vi "Unregister and Close Sessions.vi"(8 "error in":errorcluster) -> (0 "error out":errorcluster)   [LabVIEW 2020, in "VISA Measurement.lvlib"]
uses:
  VISA Measurement.lvlib
  <vilib>/MeasurementLink/MeasurementLink Session Management V1/Session Reservation/Initialize and Close Session Behavior.ctl
  <vilib>/MeasurementLink/MeasurementLink VISA/Initialize Sessions - NSess.vi
  <vilib>/MeasurementLink/MeasurementLink VISA/MeasurementLink VISA.lvlib
  <vilib>/MeasurementLink/MeasurementLink Session Management V1/Session Reservation/Session Reservation.lvclass
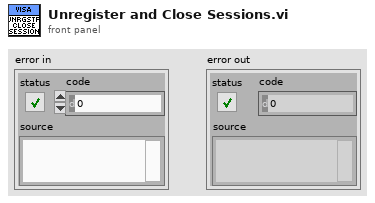
[diagram p1: front panel]
types:
  T1 = typedef "MeasurementLink Session Management V1.lvlib/Session Reservation.lvclass/Initialize and Close Session Behavior.ctl" = enum16{"Auto", "Initialize and Close", "Attach and Detach", "Initialize and Detach", "Attach and Close"}
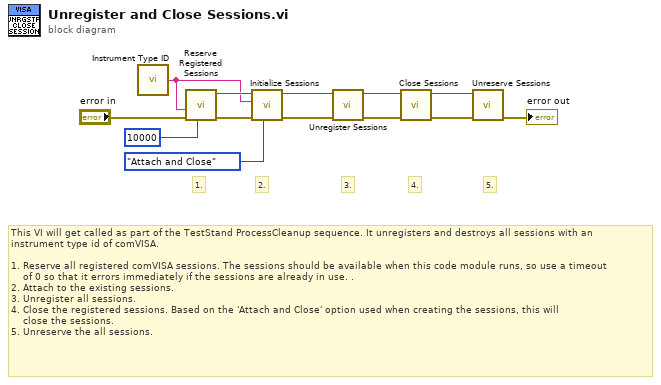
[diagram p0: block diagram]
diagram:
  # "3."
  # "5."
  # "4."
  # "2."
  # "1."
  # "This VI will get called as part of the TestStand ProcessCleanup sequence. It unregisters and destroys all sessions with an \ninstrument type id of comVISA.\n\n1. Reserve all registered comVISA sessions. The sessions should be available when this code module runs, so use a timeout\n    of 0 so that it errors immediately if the sessions are already in use. .\n2. Attach to the existing sessions.\n3. Unregister all sessions.\n4. Close the registered sessions. Based on the 'Attach and Close' option used when creating the sessions, this will\n    close the sessions.\n5. Unreserve the all sessions."
  n1 = call "Instrument Type ID.vi"() -> ("instrument type id"=w2:string)  [unwired: 5 in]
  n2 = call <vilib>:"Reserve Registered Sessions.vi"("timeout (ms)"=10000, "error in"="error in", "instrument type id"=w2) -> ("error out"=w11:errorcluster, "session reservation out"=w10:refnum<class "Session Reservation.lvclass">)  [unwired: 7 in]
  n3 = call-poly <vilib>:"Initialize Sessions.vi"("initialize and close session behavior"=Initialize_and_Close_Session_Behavior."Attach and Close", "error in"=w11, "instrument type id"=w2, "session reservation in"=w10) -> ("error out"=w7:errorcluster, "session reservation out"=w9:refnum<class "Session Reservation.lvclass">)  [unwired: 4 in, 2 out]
  n4 = call <vilib>:"Unregister Sessions.vi"("error in"=w7, "session reservation in"=w9) -> ("error out"=w4:errorcluster, "session reservation out"=w6:refnum<class "Session Reservation.lvclass">)  [unwired: 8 in]
  n5 = call <vilib>:"Close Sessions.vi"("error in"=w4, "session reservation in"=w6) -> ("error out"=w3:errorcluster, "session reservation out"=w5:refnum<class "Session Reservation.lvclass">)  [unwired: 8 in]
  n6 = call <vilib>:"Unreserve Sessions.vi"("error in"=w3, "session reservation in"=w5) -> ("error out"=→"error out":errorcluster)  [unwired: 9 in]
